vi "SUBVI1.vi"() -> ()   [LabVIEW 2022 SP3]
panel:
  in  "CLOSE":bool
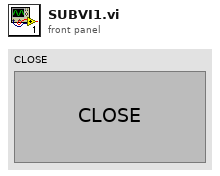
[diagram p1: front panel]
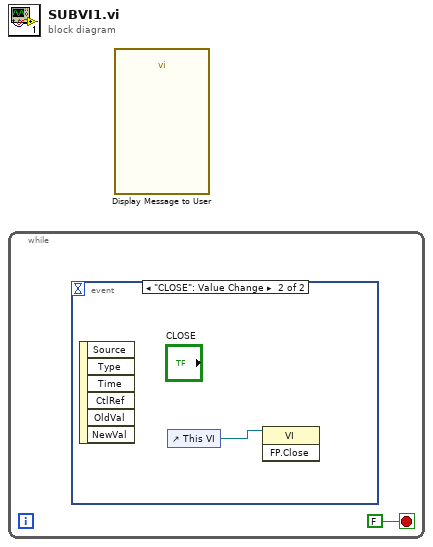
[diagram p0: block diagram]
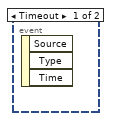
[diagram p2: hidden frame]
diagram:
  n1 = while {
    stop <- FALSE stop-if-true
    n2 = event shown="[1] \"CLOSE\": Value Change" {
      selector: _ -> [_ _]
      dyn-events: _ -> [_ _]
      timeout: _ -> [_ _]
      event Timeout {
        n3 = event-data() -> ()  [unwired: 1 in, 3 out]
      }
      event "CLOSE": Value Change {
        n4 = event-data() -> ()  [unwired: 1 in, 6 out]
        n5 = control-ref of="This VI"() -> (w2:refnum<vi>)
        n6 = invoke class="VI" method="FP.Close"(reference=w2) -> ()  [unwired: 2 in, 3 out]
      }
    }
  }
  n7 = call "Display Message to User"() -> ()  [unwired: 10 in, 2 out]
